vi "Read Text Colors.vi"(9 "Text in":refnum<class "Text.lvclass">) -> (3 "Text out":refnum<class "Text.lvclass">, 4 "Text Colors":T1)   [LabVIEW 2014, in "Raspberry Pi Compatible Compiler for LabVIEW.lvlib" / "Text.lvclass"]
uses:
  Text.lvclass
  <vilib>/Utility/miscctls.llb/LVTextColorsTypeDef.ctl
  Text.lvclass/Text.ctl
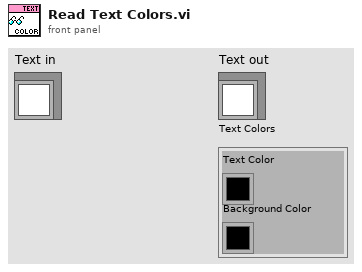
[diagram p1: front panel]
types:
  T1 = typedef "LVTextColorsTypeDef.ctl" = cluster{"Text Color":u32, "Background Color":u32}
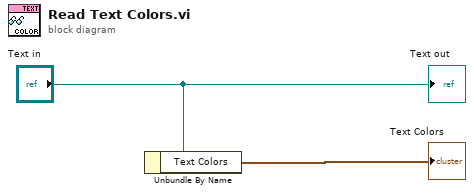
[diagram p0: block diagram]
diagram:
  n1 = Unbundle By Name("Text in") -> ("Text Colors"=→"Text Colors":T1)
  "Text out" <- "Text in"
